vi "bind text.vi"(6 "para4":u32, 7 "para3":i32, 8 "error in (no error)":errorcluster, 9 "para2":string, 10 "para1":i32, 11 "para0":dbl) -> (0 "error out":errorcluster, 2 "function return":i32, 3 "para0 out":dbl, 4 "para4 out":u32)   [LabVIEW 2020, in "sqlite3.lvlib"]
uses:
  sqlite3.lvlib
  errstr.vi
  bin/sqlite3_64.dll
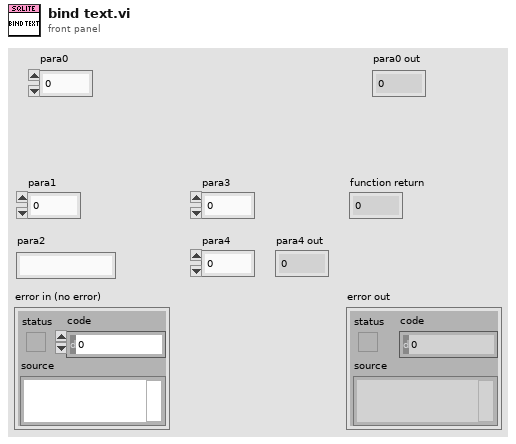
[diagram p1: front panel]
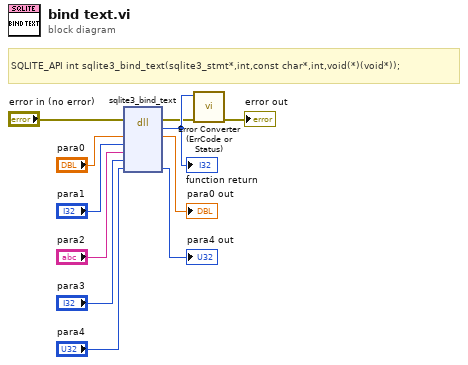
[diagram p0: block diagram]
diagram:
  # "SQLITE_API int sqlite3_bind_text(sqlite3_stmt*,int,const char*,int,void(*)(void*));"
  n1 = dll-call lib="C:/Users/Fred.Guo/Desktop/Database-configuration/externals/sqlite3/Source/bin/sqlite3_*.*" fn="sqlite3_bind_text"(error in="error in (no error)", "para0"="para0", "para1"="para1", "para2"="para2", "para3"="para3", "para4"="para4") -> (error out=w2:errorcluster, w11:i32, "para0"=→"para0 out":dbl, "para4"=→"para4 out":u32)  [unwired: 5 in, 1 out]
  "function return" <- w11
  n2 = call "Error Converter (ErrCode or Status).vi"("error in (no error)"=w2, "error code"=w11) -> ("error out"=→"error out":errorcluster)  [unwired: 9 in]
